vi "MathcadPrime2 attempt to control a variable 2.vi"() -> ()   [LabVIEW 2011]
uses:
  Variable cluster.ctl
panel:
  out "error out":errorcluster
  out "Variable Clusters out":T1
  in  "Save Worksheet":bool
  in  "stop":bool
  in  "value in":dbl
  in  "units in":string
  out "RealResult 2":dbl
  out "units 2":string
  out "SetValue":i32
  out "Array 4":string[](array[string])
  out "Array 3":dbl[](array[numeric])
  out "Array 2":errorcluster[](array[cluster])
  out "Array":string[](array[string])
  in  "MathcadPrime.IMathcadPrimeApplication2":refnum<k7>
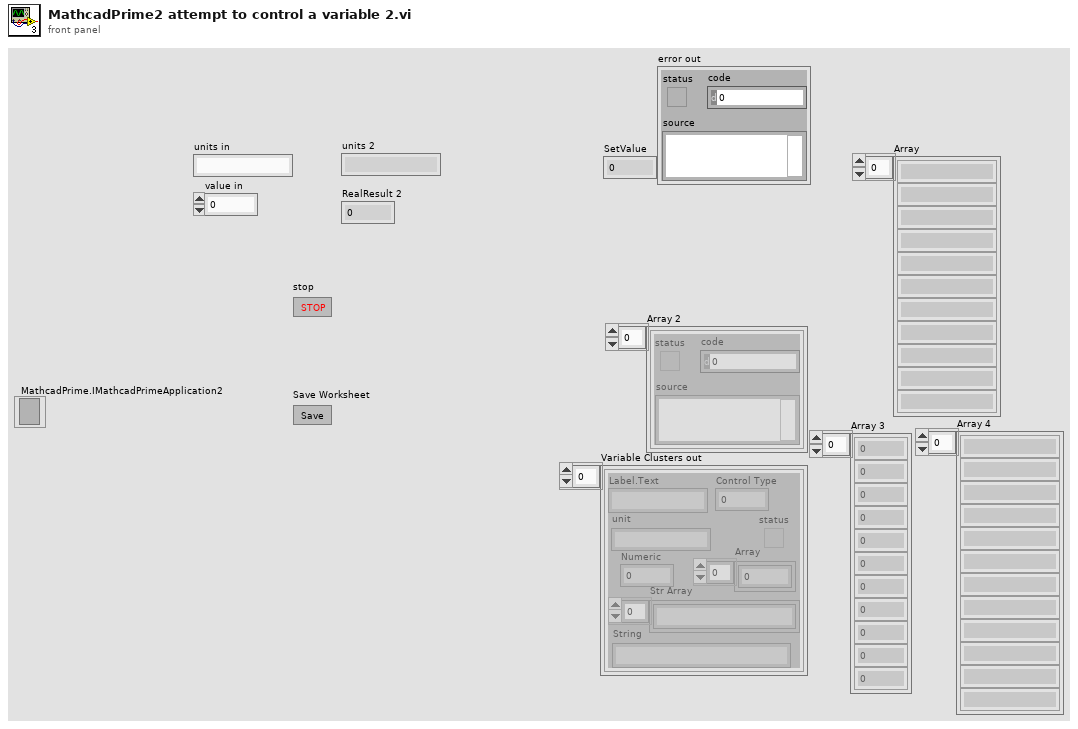
[diagram p1: front panel]
types:
  T1 = typedef "Variable cluster.ctl" = cluster{"Label.Text":string, "Control Type":u32, "Numeric":dbl, "Array":dbl[], "status":bool, "Str Array":string[], "String":string, "unit":string}[]
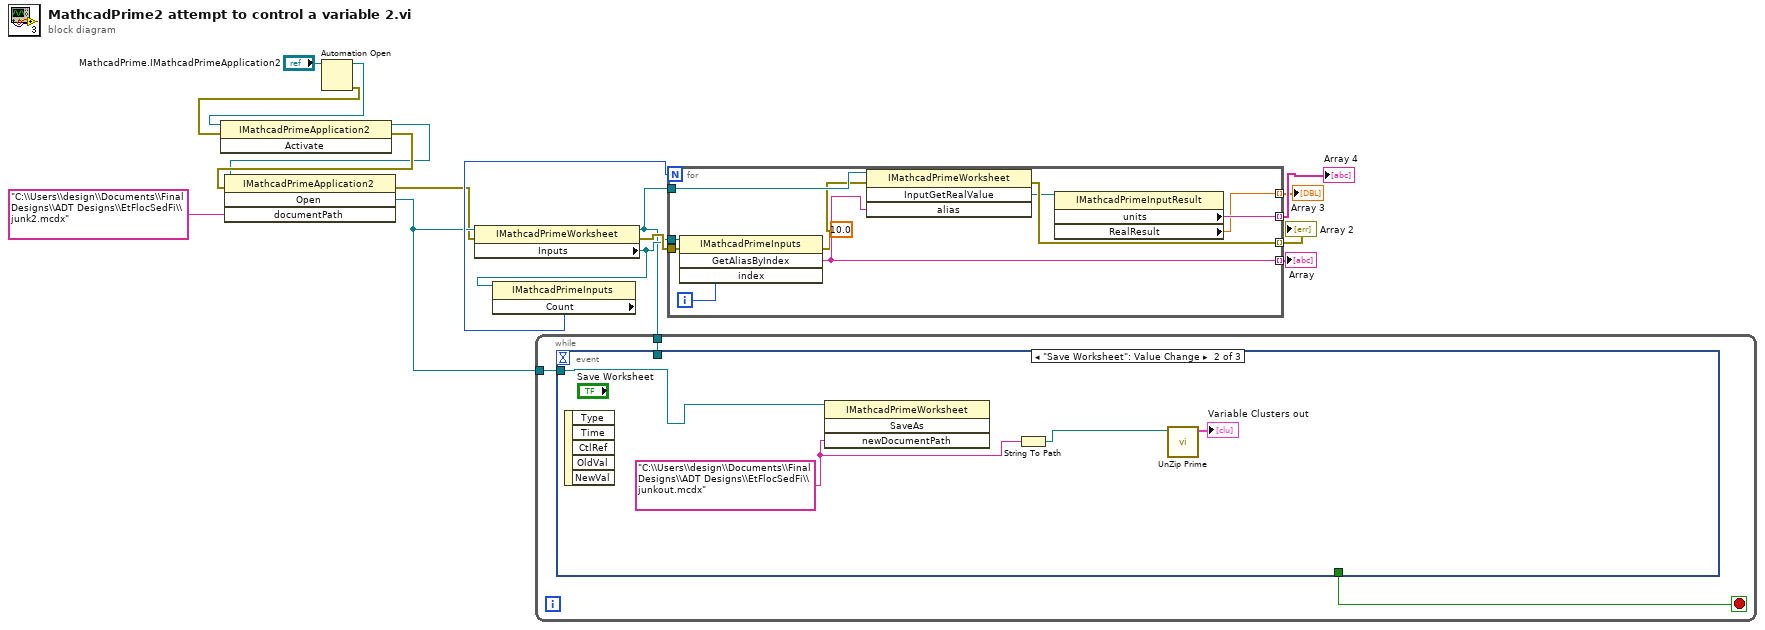
[diagram p0: block diagram]
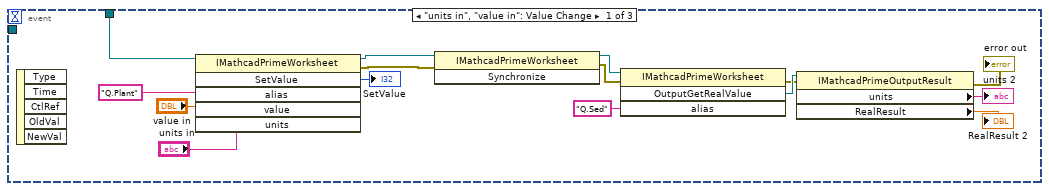
[diagram p2: hidden frame]
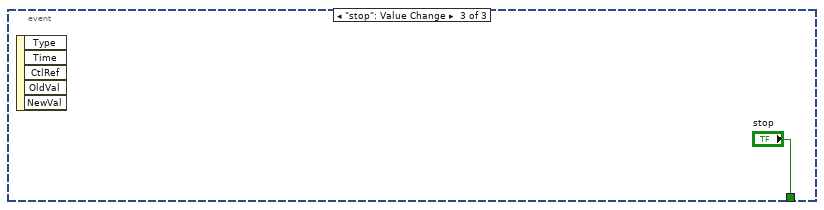
[diagram p3: hidden frame]
diagram:
  n1 = Automation Open(Automation Refnum="MathcadPrime.IMathcadPrimeApplication2") -> (Automation Refnum=w16:refnum<k7>, error out=w14:errorcluster)  [unwired: 3 in]
  n2 = invoke class="IMathcadPrimeApplication2" method="Activate"(reference=w16, error in=w14) -> (reference out=w4:refnum<k7>, error out=w15:errorcluster)  [unwired: 1 in, 1 out]
  n3 = invoke class="IMathcadPrimeApplication2" method="Open"(reference=w4, error in=w15, "documentPath"="C:\\Users\\design\\Documents\\Final Designs\\ADT Designs\\EtFlocSedFi\\junk2.mcdx") -> (error out=w2:errorcluster, "Open"=w3:refnum<k7>)  [unwired: 1 in, 2 out]
  n4 = property class="IMathcadPrimeWorksheet"(reference=w3, error in=w2) -> (reference out=w5:refnum<k7>, error out=w12:errorcluster, "Inputs"=w7:refnum<k7>)
  n5 = property class="IMathcadPrimeInputs"(reference=w7) -> ("Count"=w6:i32)  [unwired: 1 in, 2 out]
  n6 = while {
    tunnel: w5 -> [w19]
    tunnel: w3 -> [w17]
    stop <- w18 stop-if-true
    n7 = event shown="[1] \"Save Worksheet\": Value Change" {
      selector: _ -> [_ _ _]
      dyn-events: _ -> [_ _ _]
      timeout: _ -> [_ _ _]
      tunnel: w19 -> [w33 _ _]
      tunnel: [_ _ "stop"] -> w18
      tunnel: w17 -> [_ w38 _]
      event "units in", "value in": Value Change {
        n8 = event-data() -> ()  [unwired: 1 in, 5 out]
        n9 = invoke class="IMathcadPrimeWorksheet" method="SetValue"(reference=w33, "alias"="Q.Plant", "value"="value in", "units"="units in") -> (reference out=w30:refnum<k7>, error out=w23:errorcluster, "SetValue"=→"SetValue":i32)  [unwired: 2 in, 3 out]
        n10 = invoke class="IMathcadPrimeWorksheet" method="Synchronize"(reference=w30, error in=w23) -> (reference out=w29:refnum<k7>, error out=w22:errorcluster)  [unwired: 1 in, 1 out]
        n11 = invoke class="IMathcadPrimeWorksheet" method="OutputGetRealValue"(reference=w29, error in=w22, "alias"="Q.Sed") -> (error out=w21:errorcluster, "OutputGetRealValue"=w27:refnum<k7>)  [unwired: 1 in, 2 out]
        n12 = property class="IMathcadPrimeOutputResult"(reference=w27, error in=w21) -> (error out=→"error out":errorcluster, "units"=→"units 2":string, "RealResult"=→"RealResult 2":dbl)  [unwired: 1 out]
      }
      event "Save Worksheet": Value Change {
        w37 = "C:\\Users\\design\\Documents\\Final Designs\\ADT Designs\\EtFlocSedFi\\junkout.mcdx" ("documentPath")
        n13 = event-data() -> ()  [unwired: 1 in, 5 out]
        n14 = invoke class="IMathcadPrimeWorksheet" method="SaveAs"(reference=w38, "newDocumentPath"=w37) -> ()  [unwired: 2 in, 4 out]
        n15 = String To Path(string=w37) -> (path=w36:path)
        n16 = call "UnZip Prime.vi"("Path"=w36) -> ("Variable Clusters out"=→"Variable Clusters out":T1)  [unwired: 9 in, 1 out]
      }
      event "stop": Value Change {
        n17 = event-data() -> ()  [unwired: 1 in, 5 out]
      }
    }
  }
  n18 = for {
    N: w6 -> [_]
    tunnel: w12 -> [w49]
    tunnel: w7 -> [w48]
    tunnel: [w46] -> w11 mode=indexing
    tunnel: [w43] -> w10 mode=indexing
    tunnel: w5 -> [w45]
    tunnel: [w41] -> w9 mode=indexing
    tunnel: [w40] -> w8 mode=indexing
    i -> [w47]
    (unwired) 10.0 ("value")
    n19 = invoke class="IMathcadPrimeInputs" method="GetAliasByIndex"(reference=w48, error in=w49, "index"=w47) -> (error out=w44:errorcluster, "GetAliasByIndex"=w46:string)  [unwired: 1 in, 2 out]
    n20 = invoke class="IMathcadPrimeWorksheet" method="InputGetRealValue"(reference=w45, error in=w44, "alias"=w46) -> (error out=w43:errorcluster, "InputGetRealValue"=w42:refnum<k7>)  [unwired: 1 in, 2 out]
    n21 = property class="IMathcadPrimeInputResult"(reference=w42) -> ("units"=w41:string, "RealResult"=w40:dbl)  [unwired: 1 in, 2 out]
  }
  "Array" <- w11
  "Array 2" <- w10
  "Array 3" <- w8
  "Array 4" <- w9
